vi "2023_day16_Task1_with DBG.vi"() -> ()   [LabVIEW 2021]
uses:
  <vilib>/Utility/miscctls.llb/LVRowAndColumnTypeDef.ctl
  45de9bef-49e1-442e-b527-3241b48d18bf.vi
panel:
  in  "RESET TABLE":bool
  out "Table Control":string[][](table)
  out "Task 1":i32
  in  "Switch":bool caption="Ex. Data  vs.  User Data"
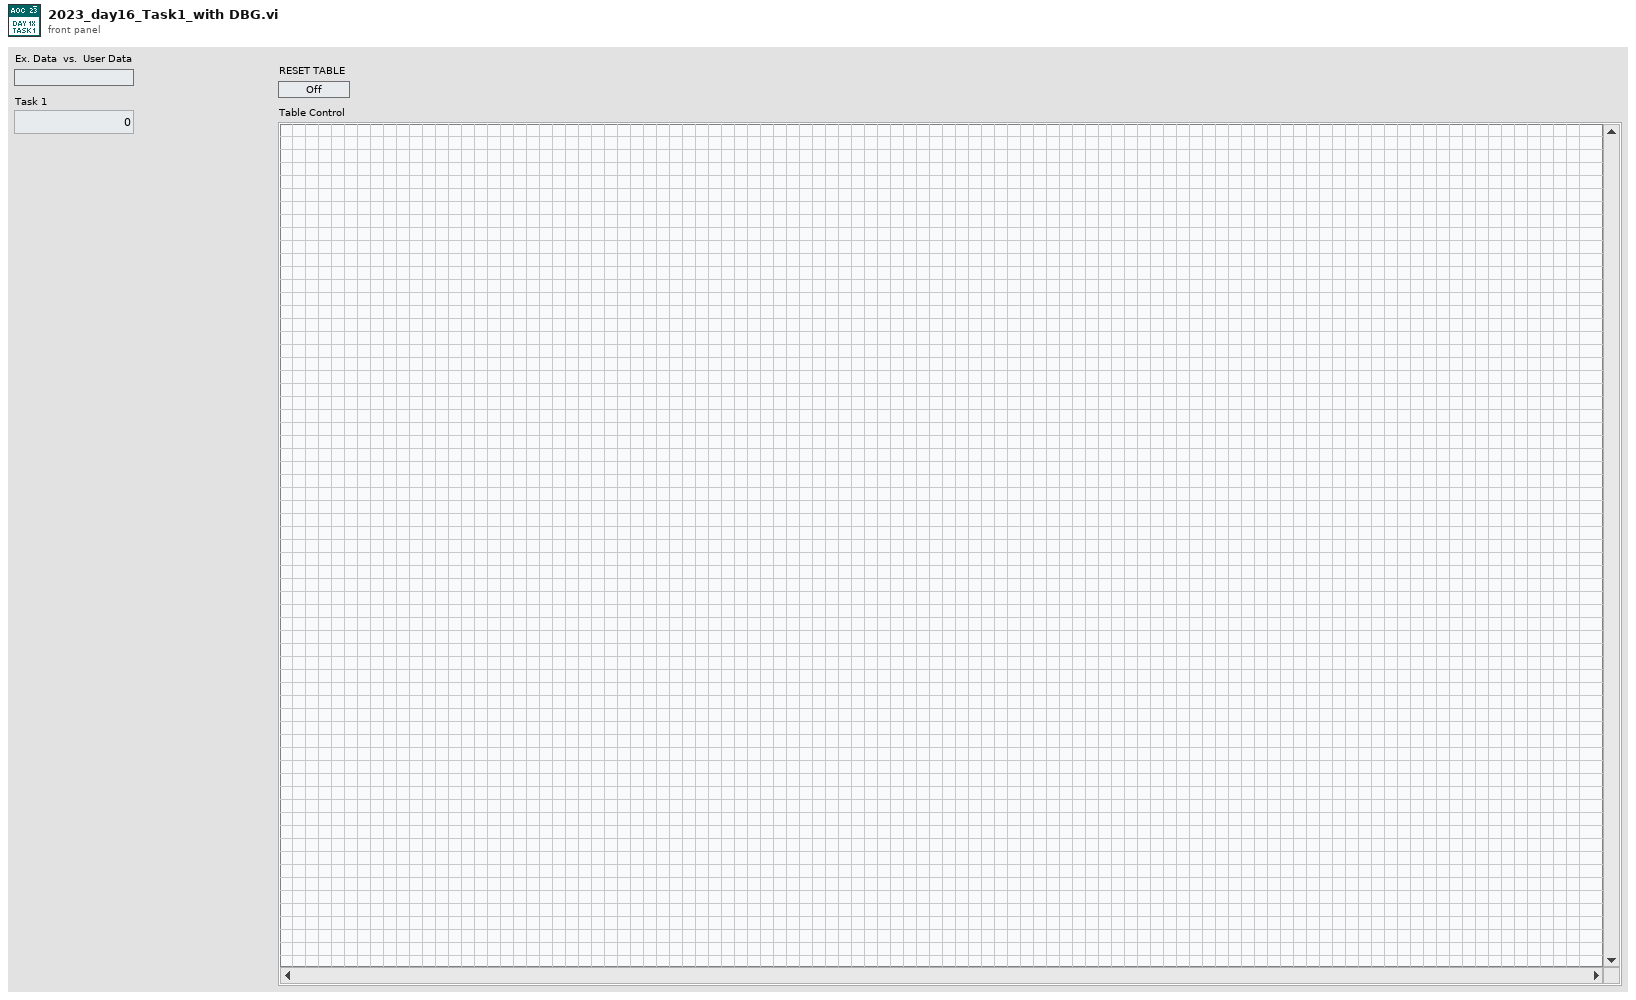
[diagram p1: front panel]
types:
  T1 = cluster{"Map":string[][], "Direction":enum16{"UP", "LEFT", "DOWN", "RIGHT"}, "Position (Row,Col)":i32[], "Energized Tiles":i32[][]}
  T2 = typedef "LVRowAndColumnTypeDef.ctl" = cluster{"Row":i32, "Column":i32}
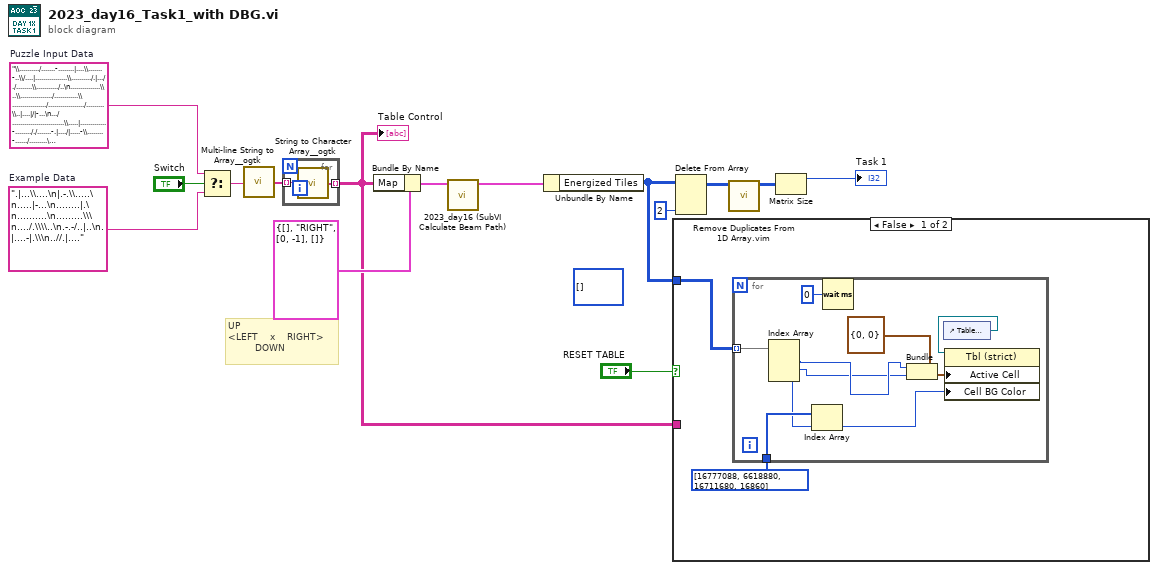
[diagram p0: block diagram]
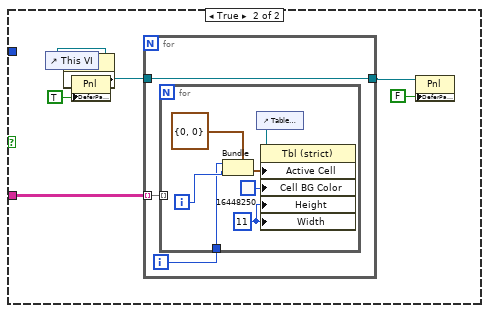
[diagram p2: hidden frame]
diagram:
  (unwired) i32[][] [] ("Energized Tiles")
  w13 = "\\........../.......-........|....\\.......-..\\/....|................\\........../.|..././........\\.........../..\n...............\\..\\................/............\\................./................../.........\\..|....|/|-...\n.../..........................\\.....|.............-.......././.......-.|..../|.....-\\........-....../.........\n|..........................-..........-......./............................-..|................-..............\n.....|......../...../.......-.\\..............................-........|............|/.../../........./........\n..\\...|..-......\\.........-\\.||........|./................\\....\\........-..\\..................../..\\....-...|.\n.|...........|............-........./.-.................|.|....../...............|..../..-..-...\\...........|.\n..............\\............................................................./......................./\\....-...\n./........|...\\.\\..|..-....\\............................|........./.................|/...............-........\n\\....\\./.............../................../....|......./........../.\\......./........-....\\......../....../|..\n./......--..........\\..|.--........-...../......./........\\.....|/..................|//...........|.........-.\n.......|.....\\-.\\..-......-.........|.....................-/\\.....-..........|.............-....\\.....\\.-.....\n..--...\\....-..|..................................-......-......\\......-................\\...../..-/....--.....\n....-.........................\\.\\............|...............|.....-...\\....|-................................\n.................-..|.\\..\\....-..........|...../.....-...-.-../.............../................-..............\n-..-......|..............................\\.....\\........|...../........\\.................../..................\n..............-.....-.|..........|.\\..................|........|...........\\.\\...|........-...................\n..\\............/...\\\\........../...-..\\.../.........\\..|................../......\\..-.../....................\\\n..................|...\\......................./...|......../..............-./...\\........\\......./|...\\..-..-.\n.................................................-................|.........................................\\.\n......-...............................|./............./...........................-\\/..../......\\..........\\..\n......\\....|..........................\\.-|..........................|....................\\.....\\/...-.........\n..\\..-|...|.....-...../......./....|...............\\................|..|.......\\...........................-..\n..\\......-.......\\.........\\................|...........|....../...../..........-./...-|..................../.\n................./.......\\...|.....\\....-................./......../..\\...........-...|.../|................\\.\n..|..\\./.........\\.\\.......................-......|....-..../.../................-.......\\../.../...../.......\n........../........./..|..-....................\\\\............\\........................-......-......|.........\n.../-....\\..\\..........\\....\\\\......................................./........\\...-.................\\.........\n................................../.................|..\\.-..|................|/....-.........................|\n...-.................||..../....................-..........................................|.-................\n..//.\\..........................|.....|-.............\\.\\......-....\\.\\.......\\............-..............\\-...\n.......|.|..-........./..|........-.....|........................-...................-......\\................-\n..-..|..........|....-.............|.|/...../../..................\\...\\................../......|....|........\n........\\..././.............../.............../....-../.....|....\\................|/.../.....|.|-..|..........\n......|..........\\...-./........-...............................\\..........|.............|..\\..|......./.....|\n.............................-................................................|................/......\\.../..-\n......-........\\..........-..../...............\\............/.....\\......|........................-.|.../.....\n...\\...............-....-........-............-...../....|.\\.../.......\\..-....................|........|.....\n.............................-...\\....|...|.......\\............................-............\\.................\n....................|...-........-.........-..\\................/....................../.|.......-.............\n......\\.........................../....-....|...........................................\\...-.........|......\\\n.............\\../\\..............|\\.\\..........|\\.../..................../\\...................|\\.......\\.......\n/.................../.\\\\.........................../...........-...-..........-..-............................\n............\\......../........-.........../........./.................-................./...........|.........\n.........\\.......|.......\\........./.....................\\..............\\\\....../...|-....\\..|..-.....|.......\n.|....-.............\\.........\\.\\../.......-...........................\\./..........................--\\......\\\n........./..../................./.................\\............................................./../.\\........\n.....-..............-.-...\\/..|....-........./.....................\\................./.\\..........-...|....|..\n........|...|.-.......|.......-............\\.../....|...\\............../............-.........................\n........................|.....\\........................./\\/.........................|.........................\n....\\..././..........|.....\\......................-................./.....|...............................|-..\n.../.........../.-......\\..../.................-...\\.....-......\\.....\\..............//.|..............-..-...\n....../............./-/.\\...........\\...\\..|/........................-...../......\\........-./\\..........||...\n.................................../............|....................../..|.....\\......\\............/.........\n.....|....\\...|.-./............................./..-....|.\\.......................-../.-..-.........\\.........\n..........\\...|../.......-|............-........../...../..........-......-../.-......|..../.-.../............\n.-.........-............|/.......-........|...................-.........-........../.-........\\..........|/...\n.........\\.........\\....../....|...\\\\......-..........-................\\................................-.....\n............-...../......|...//........\\-....|......../........./..................-................../....--.\n...............|.................................|.../...\\....................\\................|...\\.|........\n..............\\.........\\.........\\....|.-.......\\.\\........-.........../...|.....|..............\\.......\\....\n........-.-.....|.../......-\\..|.....-.........|.-................\\......./....\\...-.....\\..|/...............|\n....|.....................-...................\\......\\......-.......................-...../........./....\\....\n..|...|.......\\./..-..............\\.............................................\\../....|.....................\n..................-../........|.....-\\.../................................................./..\\...|......-...-\n.....\\......\\........\\.....................|...|../......../....../.\\........./...............................\n............../........../...........\\..\\/..|.\\...|..........-................................\\-..............\n/...............\\...|......\\............/|...................|....././...\\............................-.|.....\n...........|................/-......\\.....-.........-.............../......./............../|.................\n..-...........|..\\.............\\....|/...............|..../..............\\...............|./......|........./.\n.....\\\\..|......\\....\\.......-.................\\.-......................|........./...|.........|...|...-.....\n-...../....|....../............./.......|/../\\.............../...../-\\.../-.......|........../..............\\\\\n..........\\....................../.................|...--../..................................................\n.\\.................../......|......-.............................//......|.../|.|....\\.............\\..........\n.\\-...........-.........|..................................../........|......../...-............\\....-...-....\n......\\......|................-...../....|........-..\\.....-........//................../.....|.........-.....\n.....-..........-.|/.........-....................../......|.|./........................................./\\\\|.\n...\\................|.........../..-....|..-..........|........../....-....../......./.....-..\\.....\\\\..../...\n.....\\.....-..................-...-..../....|....|.................|...\\./.............../.......|.\\/...../...\n.||......../........../.-...|...........\\.................\\........-........|........................-...|....\n........./......\\......|...............\\.\\.................................................\\.................|\n..........................|....................|..../-...............|....|......../....-..................|..\n.-........\\.|......../...|...................|.........|............\\.....|.......\\........./.................\n................-........................\\...........|................../................-.............\\......\n.......\\..........|.............../...|.-......................../....\\.............-.......\\./...............\n..........\\...........................................-........|.......\\........./...-........\\...............\n../......./...\\|...............-........\\................./...\\...................../.....-.-....-...........-\n.\\../......../....-\\................................|.....-..|...............................-................\n..........................\\.....|................/.....\\......../.............|..............\\......./-..|....\n|.........-.|............./......-.................|.......|...\\/...........|...........................\\\\....\n-..................|.........................-.............-.....|..../.........\\...-/.....|............/\\....\n.........\\.\\....\\...........|....-.../..............|.....|-.......\\.............-......./......././.......\\..\n..../.....-...........................................\\.../..\\.|.......................-..//....-......|......\n./-..................\\..\\....................................\\......./.\\....|.................................\n...../....................................-....-/........................-/.........-.\\...|......./..-.\\......\n.....|.............-.......|-..-.................................|-...........................\\.|.....|.......\n.........\\-.............\\.............../....-....|....-.|..........\\............|.\\...|.....-................\n............/.......-....|./....|../..../......./..\\.................-..................|.....................\n../....-........./.....\\...............\\......-....|...\\........../.....|........................\\............\n...../.\\.............\\.........................-..|.......|......-......|................./......./-..........\n...\\..........\\.......................\\.-..././.........|..\\..................\\...../...|.......|............-\n........./............-..................................|.....................-..............................\n........................|.....\\.........\\..............-..\\..........||...../.\\\\./....../.....................\n.................-.............\\.../...........\\...\\......--................\\.....\\.............\\....-........\n.../-..........\\.\\............-.......-.............\\..\\.\\...../........|...-..-..|..........\\................\n\\.|..\\......\\-......./.........||..\\.........................................................-...../..........\n....|..........................................\\......-..........\\.../...\\-........|..........................\n.......-.......\\..//./....|...............\\.\\..-...\\....|....................-......\\......\\..-......../......\n/..../../....-../....-....-......................\\........./..........-/..\\......./..\\-.../..........|........\n.|....\\\\........./....\\.............-......--\\...........|.........|..\\...................../........./.\\....."  # Puzzle Input Data
  w14 = ".|...\\....\n|.-.\\.....\n.....|-...\n........|.\n..........\n.........\\\n..../.\\\\..\n.-.-/..|..\n.|....-|.\\\n..//.|...."  # Example Data
  # "UP\n<LEFT    x    RIGHT>  \n         DOWN"
  n1 = Select(t=w13, s="Switch", f=w14) -> (s? t:f=w12:string)
  n2 = call <userlib>:"Multi-line String to Array__ogtk.vi"("string"=w12) -> ("lines"=w11:string[])
  n3 = for {
    tunnel: w11 -> [w17] mode=indexing
    tunnel: [w16] -> w6 mode=indexing
    n4 = call <userlib>:"String to Character Array__ogtk.vi"("Input String"=w17) -> ("Character Array"=w16:string[])
  }
  "Table Control" <- w6
  n5 = Bundle By Name(cluster=T1 {"Map"=[], "Direction"=enum."RIGHT", "Position (Row,Col)"=[0, -1], "Energized Tiles"=[]} ("Beam"), "Map"=w6) -> (w9:T1)
  n6 = call "2023_day16 (SubVI Calculate Beam Path).vi"("Beam in"=w9) -> ("Beam out"=w8:T1)  [unwired: 10 in]
  n7 = Unbundle By Name(w8) -> ("Energized Tiles"=w1:i32[][])
  n8 = case shown="False" "RESET TABLE" {
    tunnel: w6 -> [_ w30]
    tunnel: w1 -> [w18 _]
    frame False {
      n9 = for {
        tunnel: w18 -> [w26] mode=indexing
        tunnel: u32[] [16777088, 6618880, 16711680, 16860] -> [w22]
        n10 = Index Array(array=w26) -> (element #1=w25:i32, element #2=w24:i32, element #3=w21:i32)  [unwired: 3 in]
        n11 = Index Array(array=w22, index=w21) -> (element=w20:u32)
        n12 = Wait (ms)(milliseconds to wait=u32 0) -> ()  [unwired: 1 out]
        n13 = Bundle(cluster=T2 {"Row"=0, "Column"=0} ("Active Cell:Active Cell"), "Row"=w25, "Column"=w24) -> (w28:T2)
        n14 = control-ref of="Table Control"() -> (w27:refnum<vi>)
        n15 = property on="Property Node" class="Tbl (strict)"(reference=w27, "Active Cell"=w28, "Cell BG Color"=w20) -> ()  [unwired: 1 in, 2 out]
      }
    }
    frame True {
      n16 = control-ref of="This VI"() -> (w33:refnum<vi>)
      n17 = property class="VI"(reference=w33) -> ("Panel"=w36:refnum<vi>)  [unwired: 1 in, 2 out]
      n18 = property class="Pnl"(reference=w36, "DeferPanUpdts"=TRUE ("Defer Panel Updates")) -> (reference out=w35:refnum<vi>)  [unwired: 1 in, 1 out]
      n19 = for {
        tunnel: w35 -> [w38]
        tunnel: [w38] -> w34
        tunnel: w30 -> [w37] mode=indexing
        i -> [w39]
        n20 = for {
          tunnel: w39 -> [w42]
          tunnel: w37 -> [_] mode=indexing
          i -> [w43]
          w40 = u32 11 ("Active Cell:Cell Size:Width")
          n21 = Bundle(cluster=T2 {"Row"=0, "Column"=0} ("Active Cell:Active Cell"), "Row"=w42, "Column"=w43) -> (w46:T2)
          n22 = control-ref of="Table Control"() -> (w41:refnum<vi>)
          n23 = property on="Property Node" class="Tbl (strict)"(reference=w41, "Active Cell"=w46, "Cell BG Color"=u32 16448250, "Height"=w40, "Width"=w40) -> ()  [unwired: 1 in, 2 out]
        }
      }
      n24 = property class="Pnl"(reference=w34, "DeferPanUpdts"=FALSE ("Defer Panel Updates")) -> ()  [unwired: 1 in, 2 out]
    }
  }
  n25 = Delete From Array(array=w1, index (col)=2 ("disabled index (col)")) -> (array with subset deleted=w3:i32[][])  [unwired: 2 in, 1 out]
  n26 = call "Remove Duplicates From 1D Array.vim"("array"=w3) -> ("array with duplicates removed"=w5:i32[][])  [unwired: 10 in]
  n27 = Matrix Size(0:w5) -> (1:→"Task 1":i32)  [unwired: 1 out]
